vi "COMPortDetect_DelLPT1.vi"(8 "error in":errorcluster) -> (0 "error out":errorcluster, 2 "VISA motion":refnum<visa-resource-name>, 3 "VISA laser":refnum<visa-resource-name>, 5 "Motion Find?":bool, 7 "Laser Find?":bool)   [LabVIEW 2019]
uses:
  <vilib>/Instr/_visa.llb/VISA Find Search Mode.ctl
  <vilib>/Instr/_visa.llb/VISA Configure Serial Port (Instr).vi
panel:
  out "find list":string[](array[string])
  out "Description":string[](array[string])
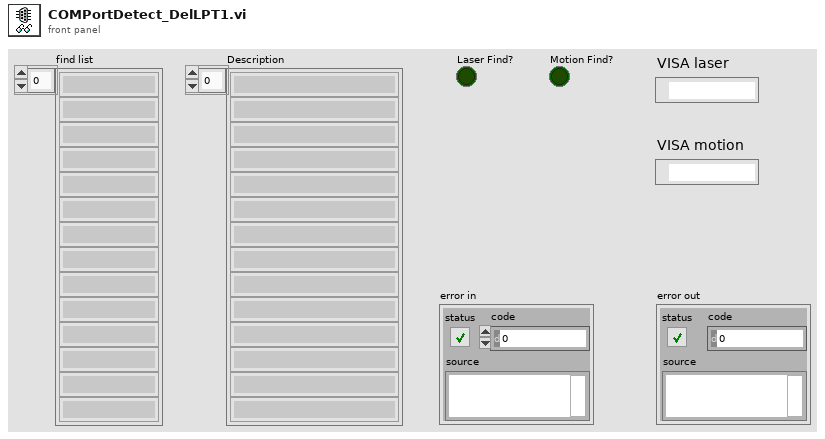
[diagram p1: front panel]
types:
  T1 = typedef "VISA Find Search Mode.ctl" = u32
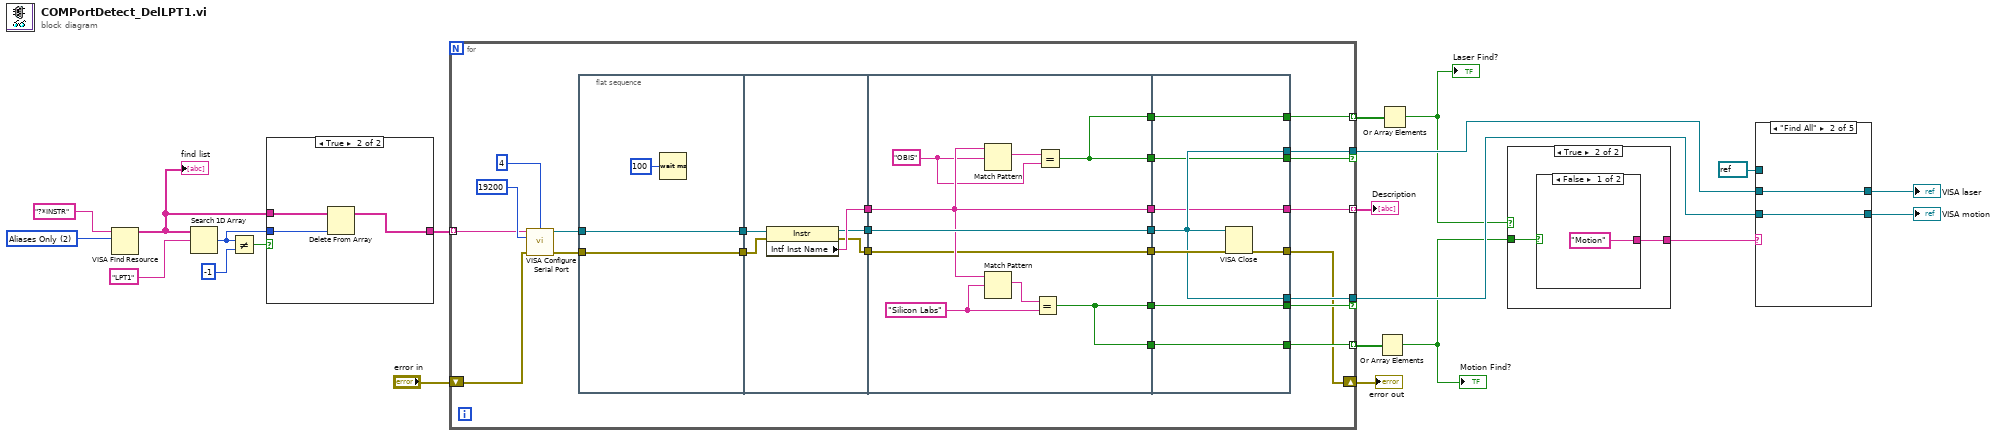
[diagram p0: block diagram]
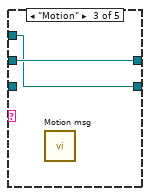
[diagram p4: hidden frame]
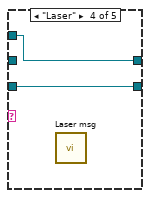
[diagram p5: hidden frame]
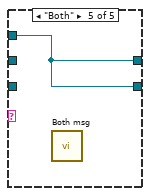
[diagram p6: hidden frame]
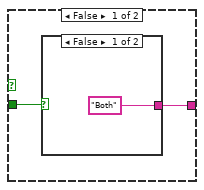
[diagram p7: hidden frame]
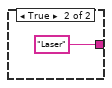
[diagram p8: hidden frame]
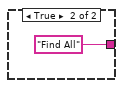
[diagram p9: hidden frame]
diagram:
  w20 = T1 2 items=["Canonical Names Only"=0, "Aliases Only"=2, "Include Matching Aliases"=3, "Include All Aliases"=4] ("Search Mode")
  n1 = VISA Find Resource(10:w20, 11:"?*INSTR" ("expression (\"?*\")")) -> (3:w5:string[])  [unwired: 1 in, 2 out]
  "find list" <- w5
  n2 = Search 1D Array(1D array=w5, element="LPT1") -> (index of element=w3:i32)  [unwired: 1 in]
  n3 = Not Equal?(x=w3, y=-1) -> (x != y?=w6:bool)
  n4 = case shown="True" w6 {
    tunnel: w5 -> [w22 w25]
    tunnel: [w22 w23] -> w4
    tunnel: w3 -> [_ w24]
    frame False {
    }
    frame True {
      n5 = Delete From Array(array=w25, index=w24) -> (array with subset deleted=w23:string[])  [unwired: 1 in, 1 out]
    }
  }
  n6 = for {
    tunnel: w4 -> [w28] mode=indexing
    tunnel: [w41] -> w13 if=w36
    tunnel: [w38] -> w12 if=w34
    tunnel: [w32] -> w19 mode=indexing
    tunnel: [w30] -> w18 mode=indexing
    tunnel: [w29] -> w9 mode=indexing
    shift-right: [w27] -> w1
    shift-left: "error in" -> [w26]
    n7 = call-poly "VISA Configure Serial Port"("VISA resource name"=w28, "termination char\n(0xA = '\\n' = LF)"=u8 4 ("termination char\n(0xA = '\\n' = LF)"), "baud rate (9600)"=u32 19200, "error in (no error)"=w26) -> ("VISA resource name out"=w49:refnum<visa-resource-name>, "error out"=w48:errorcluster)  [unwired: 10 in]
    n8 = flat-sequence {
      tunnel: w48 -> [w53]
      tunnel: w49 -> [w54]
      tunnel: [w54] -> w47
      tunnel: [w53] -> w46
      tunnel: w47 -> [w59]
      tunnel: w46 -> [w58]
      tunnel: [w57] -> w45
      tunnel: [w56] -> w43
      tunnel: [w55] -> w39
      tunnel: w45 -> [w67]
      tunnel: [w67] -> w44
      tunnel: w43 -> [w68]
      tunnel: [w68] -> w42
      tunnel: [w62] -> w40
      tunnel: w39 -> [w62]
      tunnel: [w61] -> w37
      tunnel: [w60] -> w35
      tunnel: [w61] -> w33
      tunnel: [w60] -> w31
      tunnel: w44 -> [w70]
      tunnel: w42 -> [w75]
      tunnel: [w75] -> w41
      tunnel: w40 -> [w76]
      tunnel: [w75] -> w38
      tunnel: w37 -> [w74]
      tunnel: [w74] -> w36
      tunnel: w35 -> [w73]
      tunnel: [w73] -> w34
      tunnel: w33 -> [w72]
      tunnel: [w72] -> w32
      tunnel: w31 -> [w71]
      tunnel: [w71] -> w30
      tunnel: [w70] -> w29
      tunnel: [w69] -> w27
      frame #0 {
        n9 = Wait (ms)(milliseconds to wait=u32 100) -> ()  [unwired: 1 out]
      }
      frame #1 {
        n10 = property class="Instr"(reference=w59, error in=w58) -> (reference out=w56:refnum<visa-resource-name>, error out=w55:errorcluster, "Intf Inst Name"=w57:string)
      }
      frame #2 {
        w63 = "Silicon Labs" ("regular expression")
        w65 = "OBIS" ("regular expression")
        n11 = Match Pattern(string=w67, regular expression=w65) -> (match substring=w66:string)  [unwired: 1 in, 3 out]
        n12 = Match Pattern(string=w67, regular expression=w63) -> (match substring=w64:string)  [unwired: 1 in, 3 out]
        n13 = Equal?(x=w64, y=w63) -> (x = y?=w60:bool)
        n14 = Equal?(x=w66, y=w65) -> (x = y?=w61:bool)
      }
      frame #3 {
        n15 = VISA Close(VISA resource name=w75, error in (no error)=w76) -> (error out=w69:errorcluster)
      }
    }
  }
  "Description" <- w9
  "error out" <- w1
  n16 = Or Array Elements(Boolean array=w18) -> (logical OR=w10:bool)
  "Motion Find?" <- w10
  n17 = Or Array Elements(Boolean array=w19) -> (logical OR=w11:bool)
  "Laser Find?" <- w11
  n18 = case shown="True" w11 {
    tunnel: w10 -> [w78 w82]
    tunnel: [w77 w81] -> w17
    frame False {
      n19 = case shown="False" w78 {
        tunnel: ["Both" "Laser"] -> w77
        frame False {
        }
        frame True {
        }
      }
    }
    frame True {
      n20 = case shown="False" w82 {
        tunnel: ["Motion" "Find All"] -> w81
        frame False {
        }
        frame True {
        }
      }
    }
  }
  n21 = case shown="\"Find All\"" w17 {
    tunnel: w12 -> [_ w86 _ w91 _]
    tunnel: w13 -> [_ w87 w89 _ _]
    tunnel: [w85 w87 w89 w90 w92] -> w16
    tunnel: [w85 w86 w88 w91 w92] -> w15
    tunnel: refnum<visa-resource-name> refnum ("VISA laser") -> [w85 _ w88 w90 w92]
    frame Default {
    }
    frame "Find All" {
    }
    frame "Motion" {
      n22 = call "Motion msg"() -> ()  [unwired: 10 in, 2 out]
    }
    frame "Laser" {
      n23 = call "Laser msg"() -> ()  [unwired: 10 in, 2 out]
    }
    frame "Both" {
      n24 = call "Both msg"() -> ()  [unwired: 10 in, 2 out]
    }
  }
  "VISA laser" <- w16
  "VISA motion" <- w15
